vi "MenuActivation Response.vi"(8 "error in (no error)":errorcluster, 9 "Coords":T1, 10 "Menu Refnum":refnum<k9>, 11 "Editor Handler in":refnum<class "Handler 4.lvclass">) -> (0 "error out":errorcluster, 3 "Editor Handler out":refnum<class "Handler 4.lvclass">)   [LabVIEW 2015, in "Handler 4.lvclass"]
uses:
  Handler 4.lvclass
  <vilib>/Utility/miscctls.llb/LVPoint32TypeDef.ctl
  <vilib>/LIEF/Image Editor Handler/Image Editor Handler.lvclass
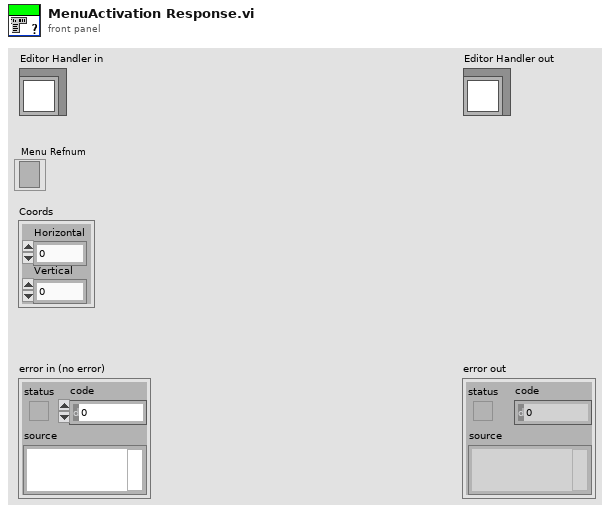
[diagram p1: front panel]
types:
  T1 = typedef "LVPoint32TypeDef.ctl" = cluster{"Horizontal":i32, "Vertical":i32}
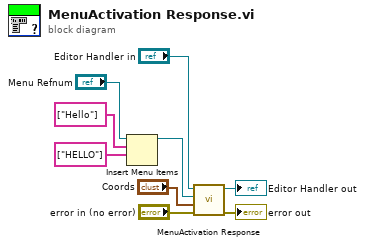
[diagram p0: block diagram]
diagram:
  n1 = Insert Menu Items(7:string[] ["HELLO"] ("item tags"), 8:string[] ["Hello"] ("item names"), 9:"Menu Refnum") -> (3:w1:refnum<k9>)  [unwired: 3 in, 2 out]
  n2 = call-parent "MenuActivation Response.vi"("error in (no error)"="error in (no error)", "Coords"="Coords", "Menu Refnum"=w1, "Editor Handler in"="Editor Handler in") -> ("error out"=→"error out":errorcluster, "Editor Handler out"=→"Editor Handler out":refnum<class "Handler 4.lvclass">)  [unwired: 6 in]
